vi "Update ROI.vi"(11 "Detail Graph in":refnum<class "Graph with Series View.lvclass">) -> (3 "Detail Graph out":refnum<class "Graph with Series View.lvclass">)   [LabVIEW 2021, in "Graph with Series View.lvclass"]
uses:
  Graph with Series View.lvclass
  Graph with Series View.lvclass/Graph with Series View.ctl
  Detail Graph/Graph with Section Views.lvclass
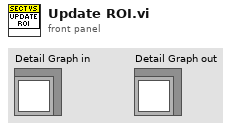
[diagram p1: front panel]
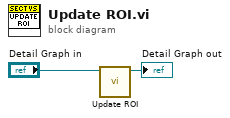
[diagram p0: block diagram]
diagram:
  n1 = call-parent "Update ROI.vi"("Detail Graph in"="Detail Graph in") -> ("Detail Graph out"=→"Detail Graph out":refnum<class "Graph with Series View.lvclass">)  [unwired: 10 in]
